vi "Check Arduino Move Complete Message.vi"() -> ()   [LabVIEW 2020]
uses:
  <vilib>/regexp/Match Regular Expression.xnode
panel:
  out "Complete?":bool
  out "m":i32
  out "position":i32
  in  "input string":string
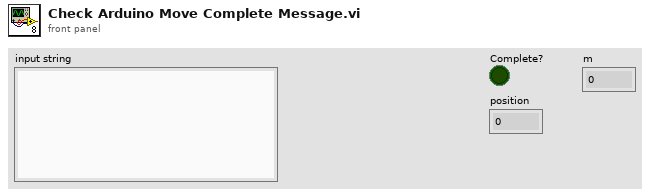
[diagram p1: front panel]
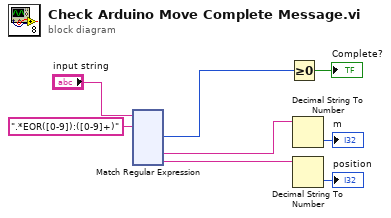
[diagram p0: block diagram]
diagram:
  n1 = xnode "Match Regular Expression"("input string"="input string", "regular expression"=".*EOR([0-9]):([0-9]+)") -> ("offset past match"=w2:i32, "submatch 1"=w4:string, "submatch 2"=w6:string)  [unwired: 4 in, 4 out]
  n2 = Greater Or Equal To 0?(x=w2) -> (x >= 0?=→"Complete?":bool)
  n3 = Decimal String To Number(string=w4) -> (number=→"m":i32)  [unwired: 2 in, 1 out]
  n4 = Decimal String To Number(string=w6) -> (number=→"position":i32)  [unwired: 2 in, 1 out]
